vi "PC main.vi"() -> ()   [LabVIEW 2020]
uses:
  <vilib>/rvi/interface/nirviMethod/nirviMethod.xnode
  <vilib>/rvi/interface/nirviReadWriteControl/nirviReadWriteControl.xnode
  <vilib>/rvi/interface/Simulation/niFpgaSimulationCallBeginRW.vi
  <vilib>/rvi/errors/niLvFpgaAdjustHostInterfaceError.vi
  <vilib>/Utility/error.llb/Error Cluster From Error Code.vi
  <vilib>/rvi/interface/nirviOpenFPGA/nirviOpenFPGA.xnode
  <vilib>/rvi/interface/nirviCloseFPGA/nirviCloseFPGA.xnode
  <vilib>/rvi/errors/niLvFpgaMergeErrorWithErrorCode.vi
  NiFpgaLv.dll
  <vilib>/FPGAPlugInAG/Dynamic/niLvFpga_Run_Dynamic.vi
  <vilib>/FPGAPlugInAG/Dynamic/niLvFpga_Reset_Dynamic.vi
  <vilib>/FPGAPlugInAG/Dynamic/niLvFpga_ConfigureFifo_Dynamic.vi
  <vilib>/LabVIEW Targets/FPGA/FlexRIO/CustomFPGAMethods/79XXR_Method_IOModuleStatusImpl.vi
  <vilib>/FPGAPlugInAG/Dynamic/niLvFpga_Close_Dynamic.vi
  <vilib>/FPGAPlugInAG/Dynamic/niLvFpga_ReadFifo_Dynamic.vi
  FPGA Bitfiles/juanmultiple_FPGATarget_FPGAmain_SDh3B+9Erj0.lvbitx
  FPGA main.vi
  <vilib>/FPGAPlugInAG/PXI-7951R/niLvFpga_Open_PXI-7951R.vi
  <vilib>/rvi/interface/common/dynamic/niFpgaDynamicAddResources.vi
panel:
  out "daq status":errorcluster
  out "Waveform Graph 2":i16[][](graph)
  out "Cumulative timeout 2":bool
  out "Instant timeout 2":bool
  in  "Delay DAQ loop by n ticks":u32
  out "Cumulative timeout":bool
  out "Instant timeout":bool
  out "Waveform Graph":i16[][](graph)
  out "loop time without delay":u32
  in  "stop":bool
  in  "Write to binary?":bool
  out "binary error status":errorcluster
  in  "Iter per file":i32
  out "running time (s)":dbl
  out "Elements Remaining":u32
  in  "max iter":i32
  out "current iter":i32
  out "Actual Depth":u32
  in  "Requested Depth":u32
  # "Attention: before starting a run, make sure you deleted the old binary files from both the folder in this folder called binaryData and the binaryData folder on the gutenberg drive, otherwise parts will get overwritten and if the old run was for a longer time, you will run into problems!"
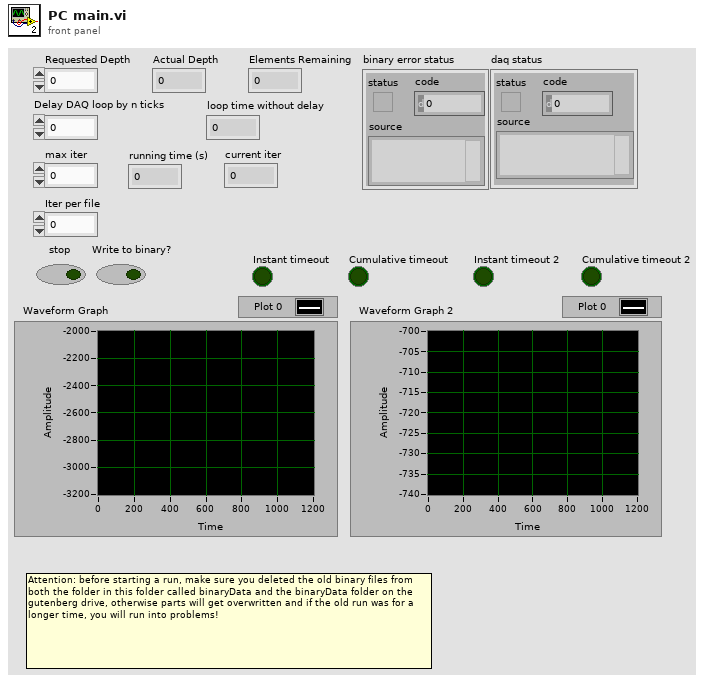
[diagram p1: front panel]
types:
  T1 = enum16{"open", "replace", "create", "open or create", "replace or create", "replace or create with confirmation"}
  T2 = enum16{"big-endian, network order", "native, host order", "little-endian"}
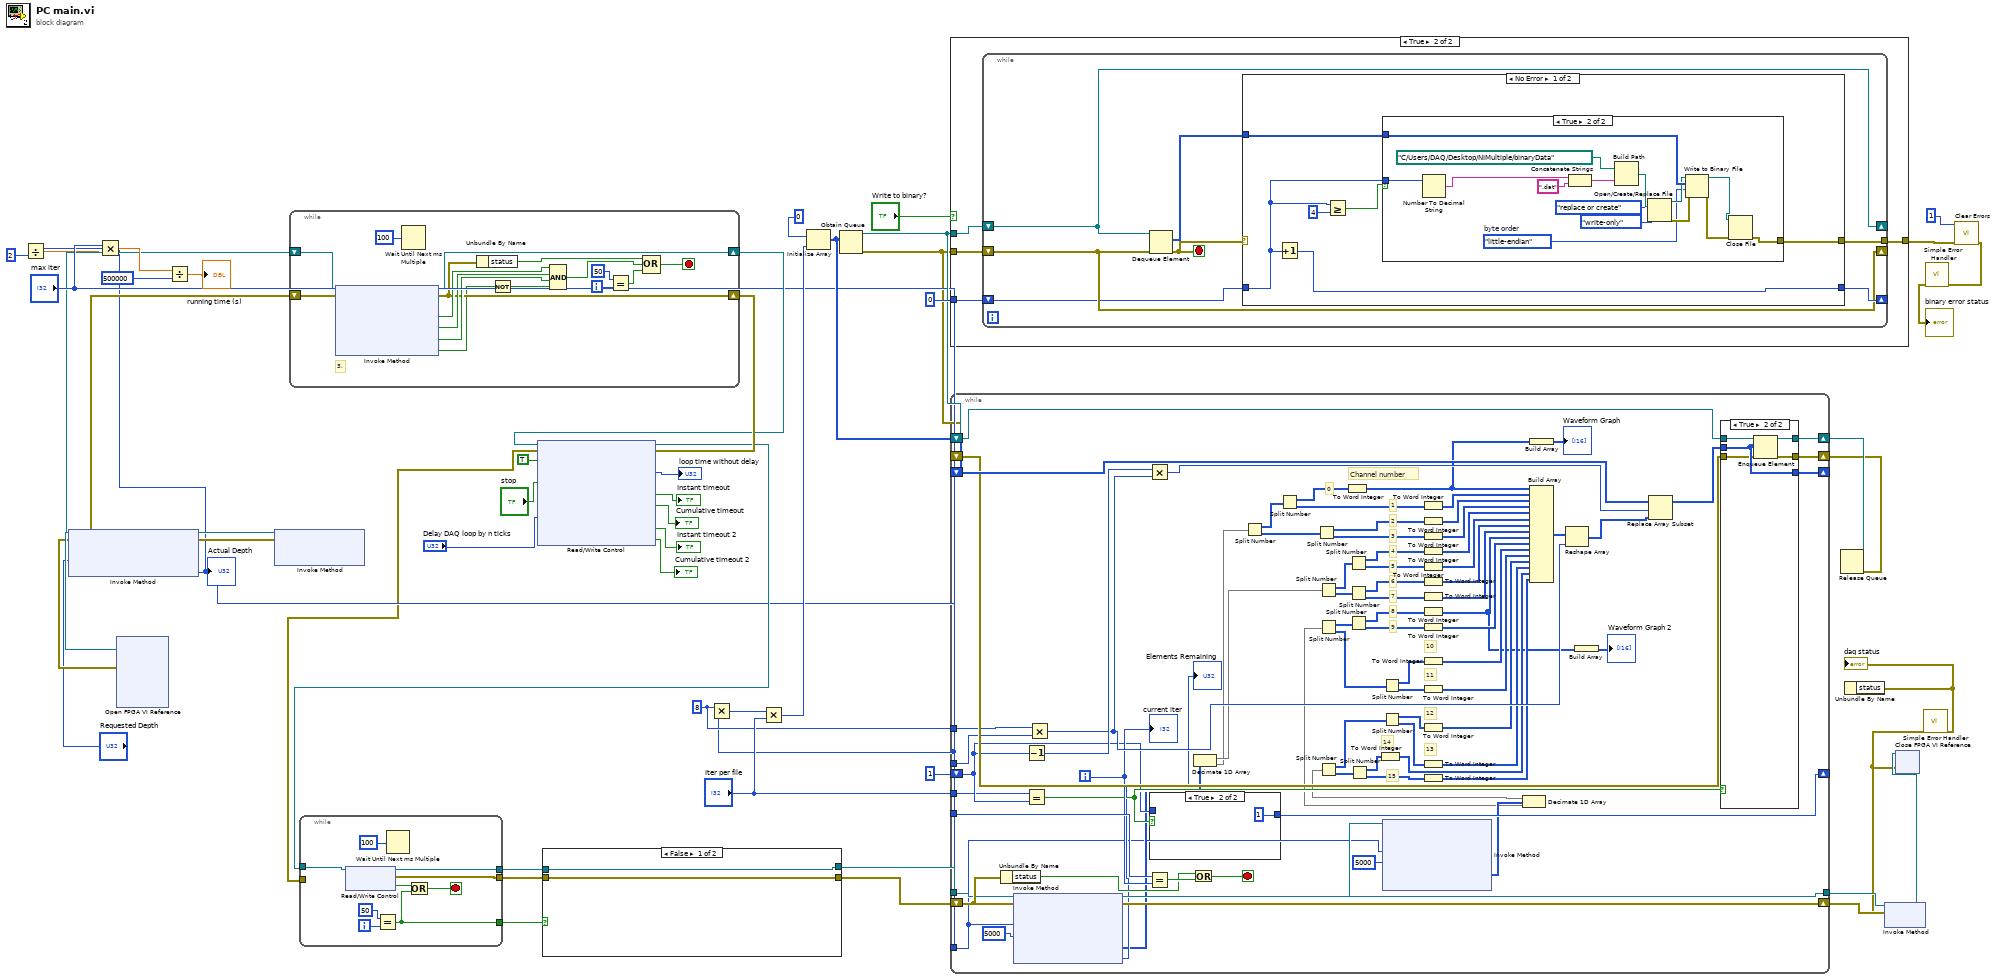
[diagram p0: block diagram]
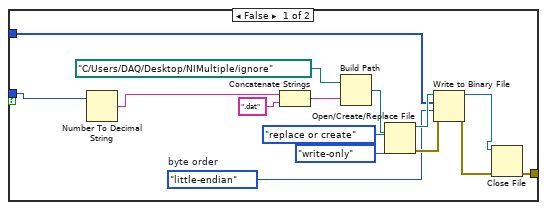
[diagram p3: hidden frame]
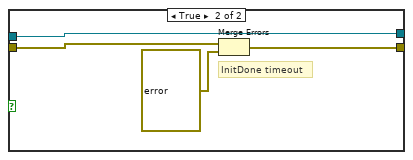
[diagram p5: hidden frame]
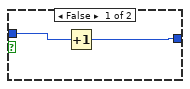
[diagram p6: hidden frame]
diagram:
  w7 = u32 8 ("x")
  n1 = xnode "Open FPGA VI Reference"() -> ("FPGA VI Reference Out"=w53:refnum<k20>, "error out"=w52:errorcluster)  [unwired: 2 in]
  n2 = xnode "Invoke Method"("FPGA VI Reference In"=w53, "error in"=w52, "Requested Depth"="Requested Depth") -> ("FPGA VI Reference Out"=w20:refnum<k20>, "error out"=w19:errorcluster, "Actual Depth"=w4:u32)
  "Actual Depth" <- w4
  n3 = Divide(x=w4, y=u32 2) -> (x/y=w5:dbl)
  n4 = Multiply(x="max iter", y=w5) -> (x*y=w45:dbl)
  n5 = Divide(x=w45, y=500000) -> (x/y=→"running time (s)":dbl)
  n6 = xnode "Invoke Method"("FPGA VI Reference In"=w20, "error in"=w19) -> ("FPGA VI Reference Out"=w18:refnum<k20>, "error out"=w17:errorcluster)  [unwired: 1 in]
  n7 = while {
    shift-right: [w60] -> w51
    shift-left: w17 -> [w68]
    shift-right: [w67] -> w50
    shift-left: w18 -> [w69]
    i -> [w62]
    stop <- w57 stop-if-true
    # "3."
    n8 = xnode "Invoke Method"("FPGA VI Reference In"=w69, "error in"=w68) -> ("FPGA VI Reference Out"=w67:refnum<k20>, "error out"=w60:errorcluster, "IO Module Present?"=w66:bool, "Power Enabled?"=w65:bool, "IO Enabled?"=w64:bool, "IO Module Mismatch?"=w55:bool)
    n9 = Wait Until Next ms Multiple(millisecond multiple=u32 100) -> ()  [unwired: 1 out]
    n10 = Unbundle By Name(w60) -> ("status"=w59:bool)
    n11 = Not(x=w55) -> (.not. x?=w54:bool)
    n12 = Compound Arithmetic op=AND(w66, w65, w64, w54) -> (w58:bool)
    n13 = Equal?(x=50, y=w62) -> (x = y?=w56:bool)
    n14 = Compound Arithmetic op=OR(w59, w58, w56) -> (w57:bool)
  }
  n15 = xnode "Read/Write Control"("FPGA VI Reference In"=w50, "error in"=w51, "Start Acquisition"=TRUE, "stop"="stop", "Delay DAQ loop by n ticks"="Delay DAQ loop by n ticks") -> ("FPGA VI Reference Out"=w37:refnum<k20>, "error out"=w1:errorcluster, "loop time"=→"loop time without delay":u32, "Instant timeout"=→"Instant timeout":bool, "Cumulative timeout"=→"Cumulative timeout":bool, "Instant timeout 2"=→"Instant timeout 2":bool, "Cumulative timeout 2"=→"Cumulative timeout 2":bool)
  n16 = while {
    tunnel: w37 -> [w78]
    tunnel: [w74] -> w39
    tunnel: [w73] -> w38
    tunnel: [w71] -> w40
    tunnel: w1 -> [_]
    i -> [w76]
    stop <- w72 stop-if-true
    n17 = xnode "Read/Write Control"("FPGA VI Reference In"=w78) -> ("FPGA VI Reference Out"=w74:refnum<k20>, "error out"=w73:errorcluster, "Init Done"=w70:bool)  [unwired: 1 in]
    n18 = Equal?(x=50, y=w76) -> (x = y?=w71:bool)
    n19 = Wait Until Next ms Multiple(millisecond multiple=u32 100) -> ()  [unwired: 1 out]
    n20 = Or(x=w70, y=w71) -> (x .or. y?=w72:bool)
  }
  n21 = case shown="False" w40 {
    tunnel: [w80 w84] -> w22
    tunnel: w39 -> [w80 w84]
    tunnel: w38 -> [w79 w82]
    tunnel: [w79 w83] -> w21
    frame False {
    }
    frame True {
      # "InitDone timeout"
      n22 = Merge Errors(w82, errorcluster {"status"=TRUE, "code"=-1, "source"="The IO Module CLIP was not ready. If you are using any external clocks, make sure they are connected and within the supported specifications."} ("error in")) -> (w83:errorcluster)
    }
  }
  n23 = Multiply(x=w7, y=w4) -> (x*y=w8:u32)
  n24 = Multiply(x=w8, y="Iter per file") -> (x*y=w46:u32)
  n25 = Initialize Array(i16 0 ("element"), w46) -> (w47:i16[])
  n26 = Obtain Queue(element data type=w47) -> (queue out=w35:refnum<queue>, error out=w32:errorcluster)  [unwired: 4 in, 1 out]
  n27 = case shown="True" "Write to binary?" {
    tunnel: 0 -> [_ w89]
    tunnel: w35 -> [_ w88]
    tunnel: w32 -> [w85 w87]
    tunnel: [w85 w86] -> w28
    frame False {
    }
    frame True {
      n28 = while {
        tunnel: [w96] -> w86
        shift-right: [w94] -> _
        shift-left: w89 -> [w91]
        shift-right: [w93] -> _
        shift-left: w88 -> [w93]
        shift-right: [w92] -> _
        shift-left: w87 -> [w92]
        stop <- w90 stop-if-true
        n29 = Dequeue Element(queue=w93, error in (no error)=w92) -> (element=w95:i16[], error out=w90:errorcluster)  [unwired: 1 in, 2 out]
        n30 = case shown="No Error" w90 {
          selector: w90 -> [_ w133]
          tunnel: [w100 w133] -> w96
          tunnel: w95 -> [w101 _]
          tunnel: w91 -> [w99 w134]
          tunnel: [w102 w134] -> w94
          frame No Error {
            n31 = Increment(x=w99) -> (x+1=w102:i32)
            n32 = Greater Or Equal?(x=w99, y=4) -> (x >= y?=w97:bool)
            n33 = case shown="True" w97 {
              tunnel: w99 -> [w105 w128]
              tunnel: w101 -> [w104 w124]
              tunnel: [w103 w118] -> w100
              frame False {
                w108 = T2."little-endian"  # byte order
                n34 = Number To Decimal String(number=w105) -> (decimal integer string=w115:string)  [unwired: 1 in]
                n35 = Concatenate Strings(w115, ".dat" ("string")) -> (w114:string)
                n36 = Build Path(base path=path "C:/Users/DAQ/Desktop/NIMultiple/ignore", name or relative path=w114) -> (appended path=w113:path)
                n37 = Open/Create/Replace File(file path (use dialog)=w113, operation (0:open)=T1."replace or create", access (0:read/write)=enum16{"read/write", "read-only", "write-only"}."write-only") -> (refnum out=w110:refnum<file>, error out=w109:errorcluster)  [unwired: 3 in, 1 out]
                n38 = Write to Binary File(file (use dialog)=w110, data=w104, error in=w109, 9:w108) -> (refnum out=w107:refnum<file>, error out=w106:errorcluster)  [unwired: 2 in, 1 out]
                n39 = Close File(refnum=w107, error in=w106) -> (error out=w103:errorcluster)  [unwired: 1 out]
              }
              frame True {
                w121 = T2."little-endian"  # byte order
                n40 = Number To Decimal String(number=w128) -> (decimal integer string=w130:string)  [unwired: 1 in]
                n41 = Concatenate Strings(w130, ".dat" ("string")) -> (w129:string)
                n42 = Build Path(base path=path "C:/Users/DAQ/Desktop/NIMultiple/binaryData", name or relative path=w129) -> (appended path=w127:path)
                n43 = Open/Create/Replace File(file path (use dialog)=w127, operation (0:open)=T1."replace or create", access (0:read/write)=enum16{"read/write", "read-only", "write-only"}."write-only") -> (refnum out=w123:refnum<file>, error out=w122:errorcluster)  [unwired: 3 in, 1 out]
                n44 = Write to Binary File(file (use dialog)=w123, data=w124, error in=w122, 9:w121) -> (refnum out=w120:refnum<file>, error out=w119:errorcluster)  [unwired: 2 in, 1 out]
                n45 = Close File(refnum=w120, error in=w119) -> (error out=w118:errorcluster)  [unwired: 1 out]
              }
            }
          }
          frame Error {
          }
        }
      }
    }
  }
  n46 = while {
    tunnel: [w213] -> w16
    tunnel: w22 -> [w142]
    shift-right: [w212] -> w15
    shift-left: w21 -> [w179]
    tunnel: w4 -> [w141]
    tunnel: "max iter" -> [w206]
    shift-right: [w201] -> _
    shift-left: w47 -> [w208]
    shift-right: [w195] -> _
    shift-left: 1 ("x") -> [w194]
    tunnel: "Iter per file" -> [w193]
    shift-right: [w192] -> w30
    shift-left: w35 -> [w199]
    shift-right: [w191] -> w29
    shift-left: w32 -> [w198]
    tunnel: w4 -> [w190]
    tunnel: w7 -> [w159]
    i -> [w197]
    stop <- w207 stop-if-true
    # "15"
    # "14"
    # "13"
    # "12"
    # "11"
    # "10"
    # "9"
    # "8"
    # "7"
    # "6"
    # "5"
    # "4"
    # "3"
    # "2"
    # "1"
    # "0"
    # "Channel number"
    n47 = Unbundle By Name(w179) -> ("status"=w210:bool)
    n48 = xnode "Invoke Method"("FPGA VI Reference In"=w142, "error in"=w179, "Number of Elements"=w141, "Timeout (ms)"=5000) -> ("FPGA VI Reference Out"=w213:refnum<k20>, "error out"=w212:errorcluster, "Data"=w182:u64[], "Elements Remaining"=→"Elements Remaining":u32)
    n49 = Decrement(x=w194) -> (x-1=w204:i32)
    n50 = Equal?(x=w193, y=w194) -> (x = y?=w196:bool)
    n51 = Multiply(x=w159, y=w190) -> (x*y=w202:u32)
    n52 = Multiply(x=w204, y=w202) -> (x*y=w205:u32)
    n53 = Equal?(x=w206, y=w197) -> (x = y?=w211:bool)
    n54 = case shown="True" w196 {
      tunnel: [w214 1 ("y")] -> w195
      tunnel: w194 -> [w215 _]
      frame False {
        n55 = Increment(x=w215) -> (x+1=w214:i32)
      }
      frame True {
      }
    }
    n56 = Or(x=w210, y=w211) -> (x .or. y?=w207:bool)
    n57 = Decimate 1D Array(w182) -> (w181:u64[], w172:u64[])
    n58 = Split Number(x=w172) -> (hi(x)=w178:u32[], lo(x)=w177:u32[])
    n59 = Split Number(x=w178) -> (hi(x)=w176:u16[], lo(x)=w175:u16[])
    n60 = Split Number(x=w177) -> (hi(x)=w174:u16[], lo(x)=w173:u16[])
    n61 = Split Number(x=w181) -> (hi(x)=w188:u32[], lo(x)=w187:u32[])
    n62 = To Word Integer(number=w176) -> (16bit integer=w158:i16[])
    n63 = Split Number(x=w188) -> (hi(x)=w186:u16[], lo(x)=w185:u16[])
    n64 = Split Number(x=w187) -> (hi(x)=w184:u16[], lo(x)=w183:u16[])
    n65 = xnode "Invoke Method"("FPGA VI Reference In"=w142, "Number of Elements"=w141, "Timeout (ms)"=5000) -> ("Data"=w139:u64[])  [unwired: 1 in, 3 out]
    n66 = To Word Integer(number=w175) -> (16bit integer=w157:i16[])
    n67 = To Word Integer(number=w174) -> (16bit integer=w156:i16[])
    n68 = To Word Integer(number=w173) -> (16bit integer=w155:i16[])
    n69 = To Word Integer(number=w186) -> (16bit integer=w154:i16[])
    n70 = To Word Integer(number=w185) -> (16bit integer=w153:i16[])
    n71 = To Word Integer(number=w184) -> (16bit integer=w152:i16[])
    n72 = To Word Integer(number=w183) -> (16bit integer=w151:i16[])
    n73 = Decimate 1D Array(w139) -> (w135:u64[], w136:u64[])
    n74 = Split Number(x=w136) -> (hi(x)=w165:u32[], lo(x)=w164:u32[])
    n75 = Split Number(x=w135) -> (hi(x)=w171:u32[], lo(x)=w170:u32[])
    n76 = Split Number(x=w165) -> (hi(x)=w163:u16[], lo(x)=w162:u16[])
    n77 = Split Number(x=w170) -> (hi(x)=w167:u16[], lo(x)=w166:u16[])
    n78 = To Word Integer(number=w167) -> (16bit integer=w145:i16[])
    n79 = Split Number(x=w164) -> (hi(x)=w161:u16[], lo(x)=w160:u16[])
    n80 = Split Number(x=w171) -> (hi(x)=w169:u16[], lo(x)=w168:u16[])
    n81 = To Word Integer(number=w163) -> (16bit integer=w138:i16[])
    n82 = To Word Integer(number=w162) -> (16bit integer=w150:i16[])
    n83 = To Word Integer(number=w161) -> (16bit integer=w149:i16[])
    n84 = To Word Integer(number=w160) -> (16bit integer=w148:i16[])
    n85 = To Word Integer(number=w169) -> (16bit integer=w147:i16[])
    n86 = To Word Integer(number=w168) -> (16bit integer=w146:i16[])
    n87 = To Word Integer(number=w166) -> (16bit integer=w144:i16[])
    n88 = Build Array(w158) -> (→"Waveform Graph":i16[][])
    n89 = Build Array(w158, w157, w156, w155, w154, w153, w152, w151, w138, w150, w149, w148, w147, w146, w145, w144) -> (w143:i16[][])
    n90 = Reshape Array(w143, w202) -> (w203:i16[])
    n91 = Build Array(w138) -> (→"Waveform Graph 2":i16[][])
    n92 = Replace Array Subset(array=w208, new element=w203, index=w205) -> (w200:i16[])
    n93 = case shown="True" w196 {
      tunnel: [w219 w224] -> w201
      tunnel: w200 -> [w219 w224]
      tunnel: w199 -> [w217 w223]
      tunnel: w198 -> [w218 w222]
      tunnel: [w217 w221] -> w192
      tunnel: [w218 w220] -> w191
      frame False {
      }
      frame True {
        n94 = Enqueue Element(queue=w223, element=w224, error in (no error)=w222) -> (queue out=w221:refnum<queue>, error out=w220:errorcluster)  [unwired: 1 in, 1 out]
      }
    }
    "current iter" <- w197
  }
  n95 = Release Queue(queue=w30, error in (no error)=w29) -> ()  [unwired: 1 in, 3 out]
  n96 = xnode "Invoke Method"("FPGA VI Reference In"=w16, "error in"=w15) -> ("FPGA VI Reference Out"=w14:refnum<k20>, "error out"=w2:errorcluster)
  n97 = xnode "Close FPGA VI Reference"("FPGA VI Reference In"=w14, "error in"=w2) -> ()  [unwired: 1 out]
  n98 = call <vilib>:"Simple Error Handler.vi"("error in (no error)"=w2) -> ("error out"=w3:errorcluster)  [unwired: 1 in, 7 out]
  "daq status" <- w3
  n99 = Unbundle By Name(w3) -> ()  [unwired: 1 out]
  n100 = call <vilib>:"Clear Errors.vi"("error in (no error)"=w28, "specific error code to clear (0: all)"=1) -> ("error out"=w27:errorcluster)  [unwired: 4 in, 1 out]
  n101 = call <vilib>:"Simple Error Handler.vi"("error in (no error)"=w27) -> ("error out"=→"binary error status":errorcluster)  [unwired: 1 in, 7 out]
